vi "GameEngine.vi"(6 "ImagesFolder":path, 7 "IterationDelay (ms)":u32=10, 8 "error in (no error)":errorcluster, 9 "Player2":refnum<class "Player.lvclass">, 10 "Player1":refnum<class "Player.lvclass">, 11 "Board":refnum<class "Board.lvclass">) -> (0 "error out":errorcluster, 2 "GameRecord":refnum<class "GameRecorder.lvclass">, 3 "GameResult":T1)   [LabVIEW 2015, in "TronviewGame.lvlib"]
uses:
  TronviewGame.lvlib
  Game/GameResult.ctl
  Board/Board.lvclass
  Player/Player.lvclass
  GameRecorder/GameRecorder.lvclass
  Game/Game.lvclass/Game.ctl
  Game/GetGameRecorder.vi
  Game/Game.lvclass
  TronviewPresentation/BoardDisplay/BoardDisplay.lvclass
panel:
  out "Board":picture[][](array[picture])
  out "Finished?":bool
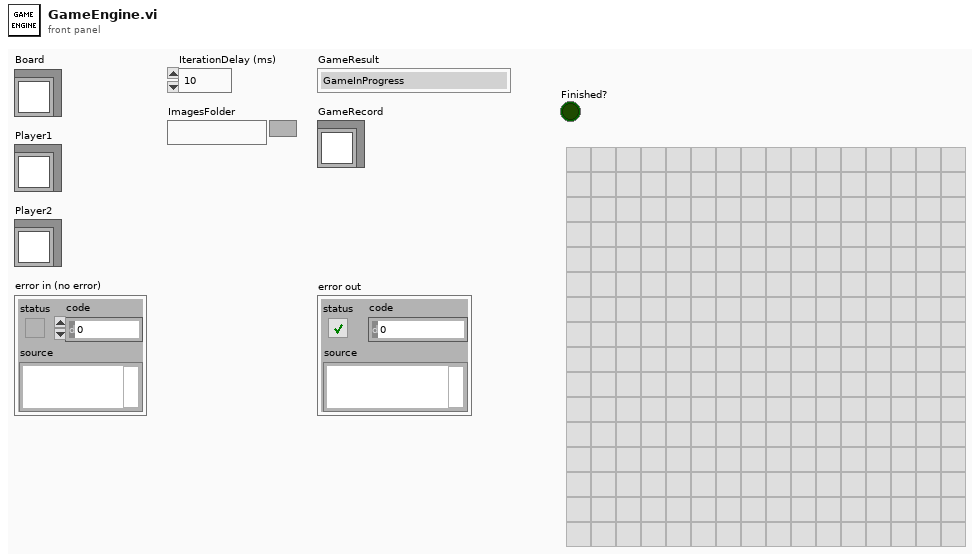
[diagram p1: front panel]
types:
  T1 = typedef "TronviewGame.lvlib/Game.lvclass/GameResult.ctl" = enum16{"GameInProgress", "Draw", "Player1Won", "Player2Won"}
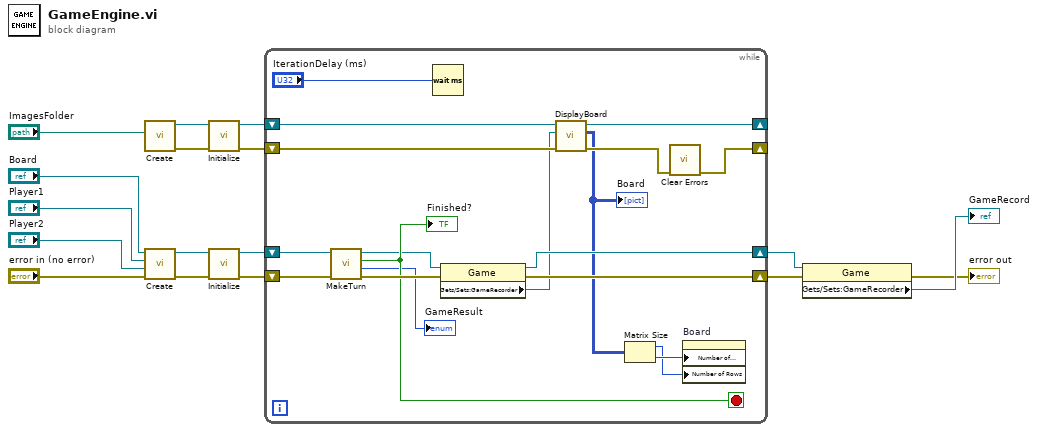
[diagram p0: block diagram]
diagram:
  n1 = call "Create.vi"("ImagesFolder"="ImagesFolder") -> ("error out"=w4:errorcluster, "BoardDisplay out"=w5:refnum<class "BoardDisplay.lvclass">)  [unwired: 9 in]
  n2 = call "Create.vi"("error in (no error)"="error in (no error)", "Player2"="Player2", "Player1"="Player1", "Board"="Board") -> ("error out"=w16:errorcluster, "Game out"=w17:refnum<class "Game.lvclass">)  [unwired: 6 in]
  n3 = call "Initialize.vi"("error in (no error)"=w4, "BoardDisplay in"=w5) -> ("error out"=w2:errorcluster, "BoardDisplay out"=w1:refnum<class "BoardDisplay.lvclass">)  [unwired: 8 in]
  n4 = call "Initialize.vi"("error in (no error)"=w16, "Game in"=w17) -> ("error out"=w14:errorcluster, "Game out"=w15:refnum<class "Game.lvclass">)  [unwired: 8 in]
  n5 = while {
    shift-right: [w21] -> w12
    shift-left: w15 -> [w35]
    shift-right: [w23] -> w13
    shift-left: w14 -> [w34]
    shift-right: [w24] -> _
    shift-left: w1 -> [w27]
    shift-right: [w18] -> _
    shift-left: w2 -> [w26]
    stop <- w31 stop-if-true
    n6 = call "MakeTurn.vi"("error in (no error)"=w34, "Game in"=w35) -> ("error out"=w33:errorcluster, "GameResult"=→"GameResult":T1, "Finished?"=w31:bool, "Game out"=w22:refnum<class "Game.lvclass">)  [unwired: 6 in]
    "Finished?" <- w31
    n7 = Wait (ms)(milliseconds to wait="IterationDelay (ms)") -> ()  [unwired: 1 out]
    n8 = property class="Game"(reference=w22, error in=w33) -> (reference out=w21:refnum<class "Game.lvclass">, error out=w23:errorcluster, "Gets/Sets:GameRecorder"=w20:refnum<class "GameRecorder.lvclass">)
    n9 = call "DisplayBoard.vi"("error in (no error)"=w26, "GameRecorder"=w20, "BoardDisplay in"=w27) -> ("error out"=w25:errorcluster, "BoardVisulalization"=w19:picture[][], "BoardDisplay out"=w24:refnum<class "BoardDisplay.lvclass">)  [unwired: 6 in]
    "Board" <- w19
    n10 = Matrix Size(0:w19) -> (1:w28:i32, 2:w29:i32)
    n11 = call <vilib>:"Clear Errors.vi"("error in (no error)"=w25) -> ("error out"=w18:errorcluster)  [unwired: 5 in, 1 out]
    n12 = property on="Board" class="Arr (strict)"("Number of Columns"=w29, "Number of Rows"=w28) -> ()  [unwired: 2 in, 2 out]
  }
  n13 = property class="Game"(reference=w12, error in=w13) -> (error out=→"error out":errorcluster, "Gets/Sets:GameRecorder"=→"GameRecord":refnum<class "GameRecorder.lvclass">)  [unwired: 1 out]
